vi "EV Rotator Control Editor.vi"(6 "Channel":i32=1, 8 "Calibration in":string, 9 "Hardware in":string, 10 "Setup in":string, 11 "Editor seq info":T1 {"Steps config"."Loop Info"."unit scale" items=["Log", "Lin"]; "Steps config"."Loop Info"."unit dB ref" format="%#_6p"}) -> (1 "Step name out":string="Calibration Default", 2 "Setup out":string, 3 "Sequence channels & curves out":string[](array[string]))   [LabVIEW 2012]
uses:
  custom and SC Run Seq Sub VIs.llb/editor seq info.ctl
  custom and SC Run Seq Sub VIs.llb/Steps config.ctl
panel:
  in  "Absolute mode":bool
  in  "Port name":string
  in  "Function to run":enum16{"Home", "MoveDegrees"}(ring)
  in  "Vertical angle":dbl format="%.3f"
  in  "Horizontal angle":dbl format="%.3f"
  in  "Save as":bool
  in  "save":bool
  in  "revert":bool
  in  "continue loop?":bool
  in  "cancel":bool
  in  "load":bool
  # "Reminder:  You must edit this custom step from\nwithin a sequence for it to remember your settings."
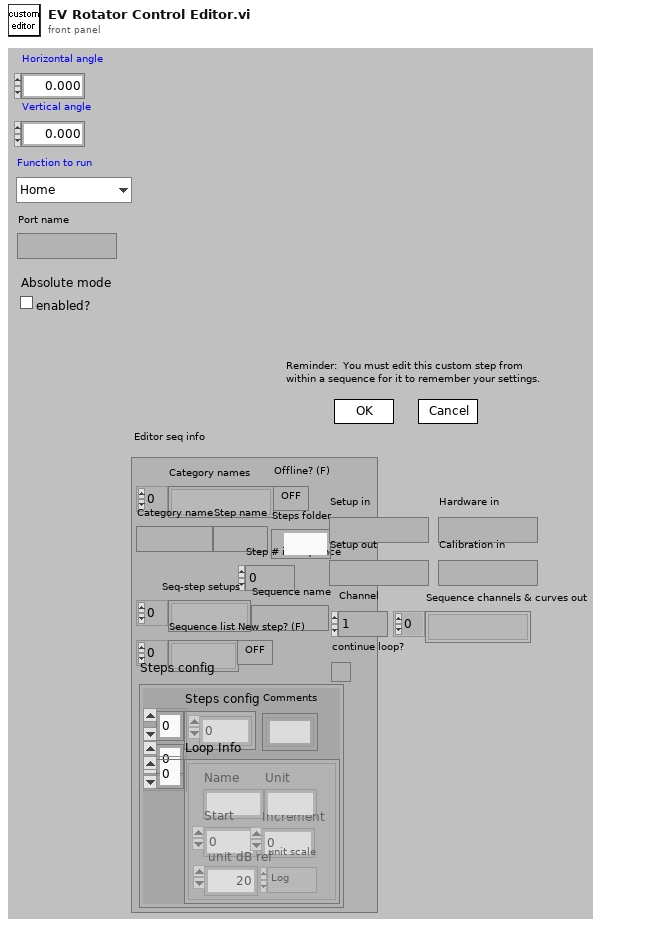
[diagram p1: front panel]
types:
  T1 = typedef "editor seq info.ctl" = cluster{"Category names":string[], "Category name":string, "Step name":string, "Step # in sequence":i32, "Seq-step setups":string[], "Sequence name":string, "Sequence list":string[], "New step? (F)":bool, "Steps config":T2, "Offline? (F)":bool, "Steps folder":path}
  T2 = typedef "Steps config.ctl" = cluster{"Steps config":i32[][], "Loop Info":cluster{"Name":string, "Start":dbl, "Increment":dbl, "Unit":string, "unit dB ref":dbl, "unit scale":u16}[], "Comments":string[]}
  T3 = cluster{"Horizontal angle":dbl, "Vertical angle":dbl, "FunctionToRun":enum16{"Home", "MoveDegrees"}, "Port name":string, "Absolute position mode":bool}
  T4 = cluster{"load":bool, "revert":bool, bool, "cancel":bool, "Save as":bool, bool, bool}
  T5 = cluster{"load":bool, "revert":bool, "save":bool, "cancel":bool, "Save as":bool, "close panel":bool, "apply":bool}
  T6 = typedef "seq step setup.ctl" = cluster{"Input Signal Channels":i32[], "Output Signal Channels":i32[], "Curves selected":string[][], "Curves generated":string[], "Step setup flat":string, "Trigger Signal Channel":i32, "Curves Generated Assumptions":cluster{"seq-setup in":string, "Relevant subset of mem list Grouping":cluster{T7[]}[]}}
  T7 = typedef "Memory List Grouping.ctl" = cluster{"item name":string, "parent":string, "Open?":bool, "Type":enum16{"item", "custom group", "auto group"}}
  T8 = typedef "data cluster.ctl" = cluster{"Name":string, "Curve":cluster{"x":dbl, "y":dbl, "z":dbl}[], "X data":T9, "Y data":T9, "Z data":T9, "X axis":u16, "Y axis":u16, "Z axis":u16, "X unit":string, "Y unit":string, "Z unit":string, "X dB ref":dbl, "Y dB ref":dbl, "Z dB ref":dbl, "single val":bool, "protected":bool, "display X":bool, "display Y":bool, "display Z":bool, "Plot Settings":cluster{"Color":u32, "Interpolation":u8, "Point Style":u8, "Line Style":u8, "Point Color":u32, "Line Width":u8, "Bar Plot Style":u8, "Fill To":i16}, "Test Info":string}
  T9 = typedef "Axis Unit Type.ctl" = u16
  T10 = typedef "waveform cluster.ctl" = cluster{"Name":string, "Waveform":cluster{"X0":dbl, "dX":dbl, "Y":sgl[]}, "X data":T9, "Y data":T9, "Y axis":T9, "X unit":string, "Y unit":string, "Y dB ref":dbl, "display Y":bool, "display X":bool, "Overload?":bool, "protected":bool, "Sqc history":string[], "Signal Channel ID":i32, "Plot Settings":cluster{"Color":u32, "Interpolation":u8, "Point Style":u8, "Line Style":u8, "Point Color":u32, "Line Width":u8, "Bar Plot Style":u8, "Fill To":i16}, "Test Info":string}
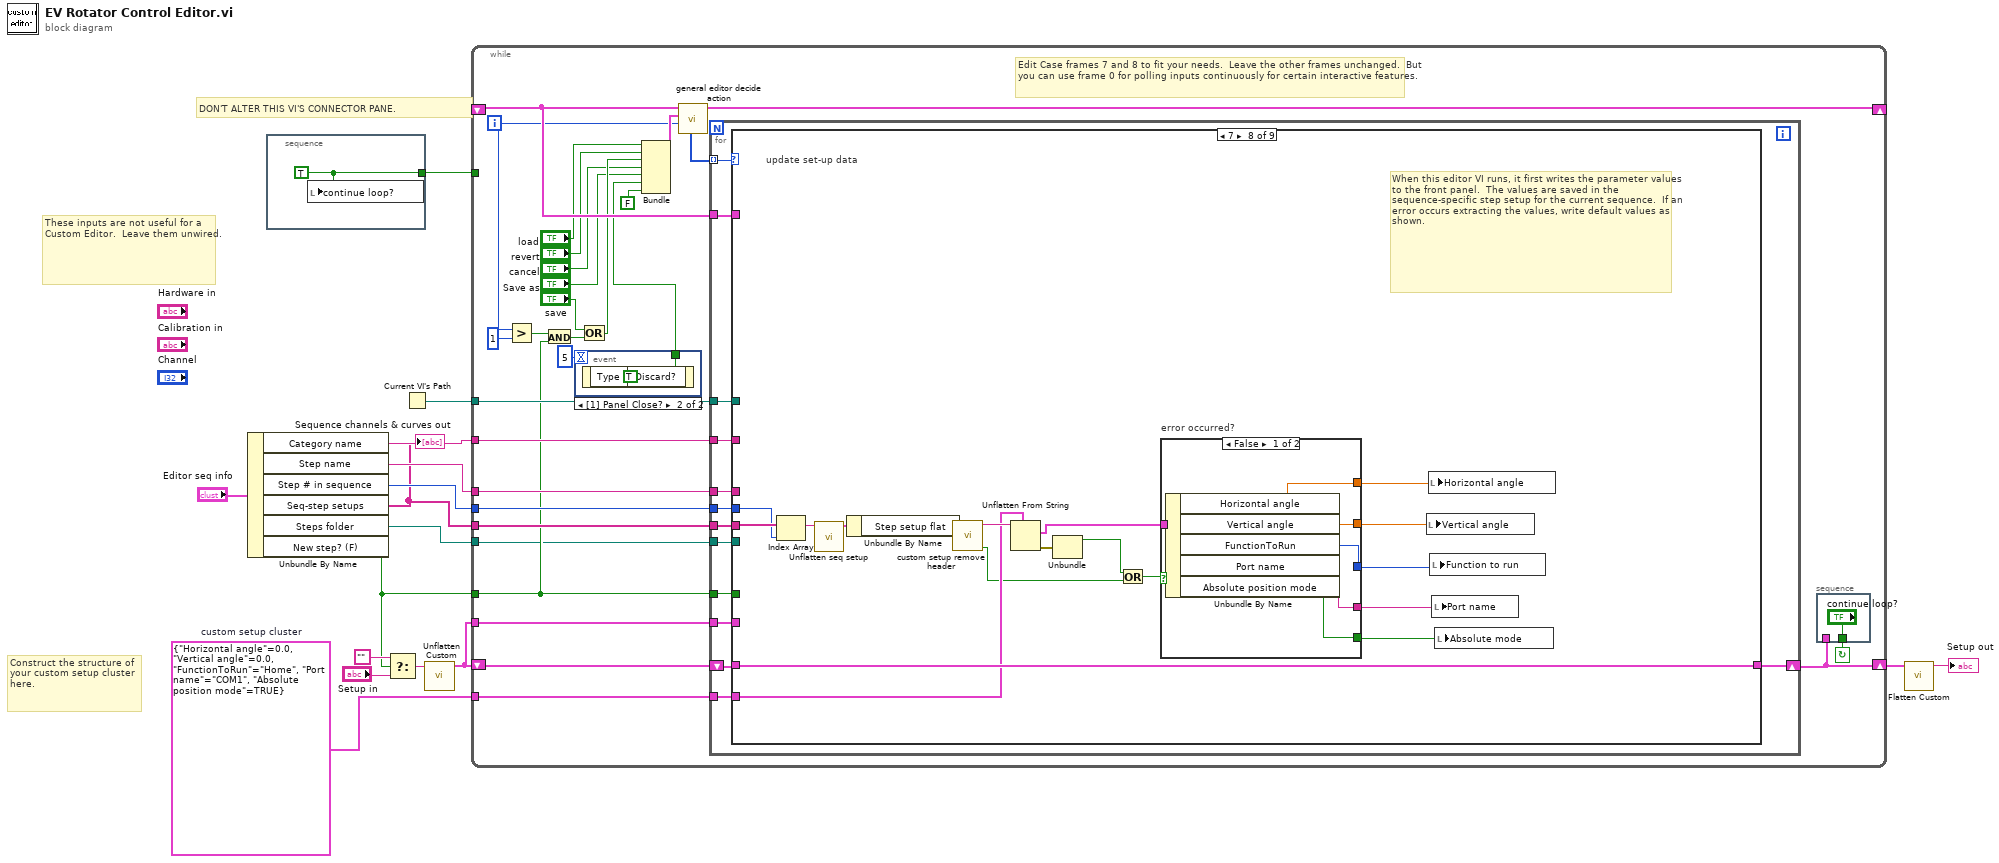
[diagram p0: block diagram]
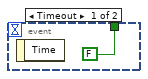
[diagram p2: hidden frame]
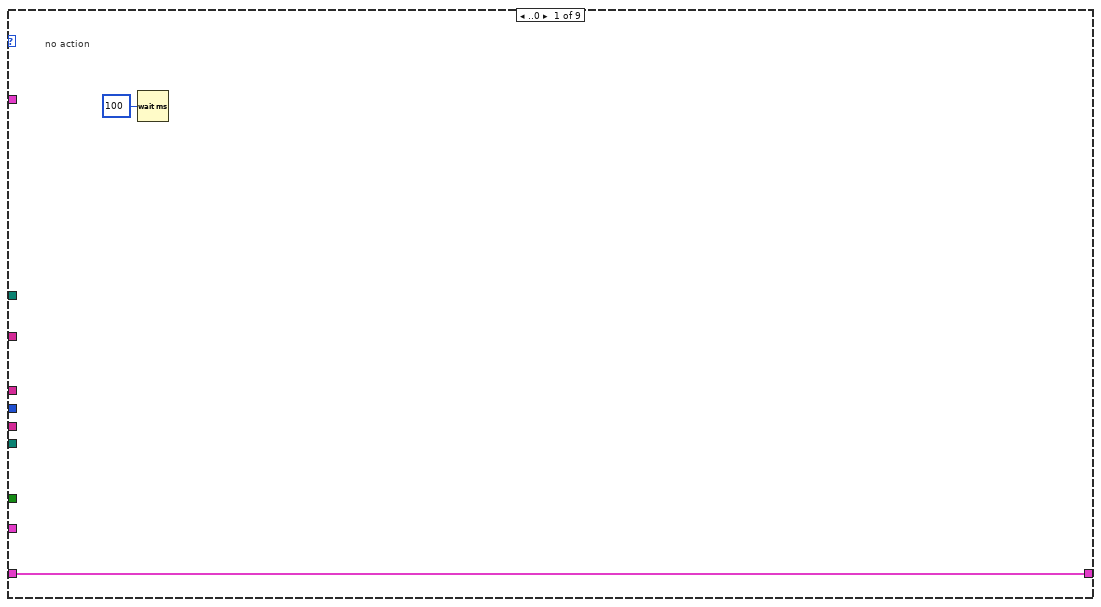
[diagram p3: hidden frame]
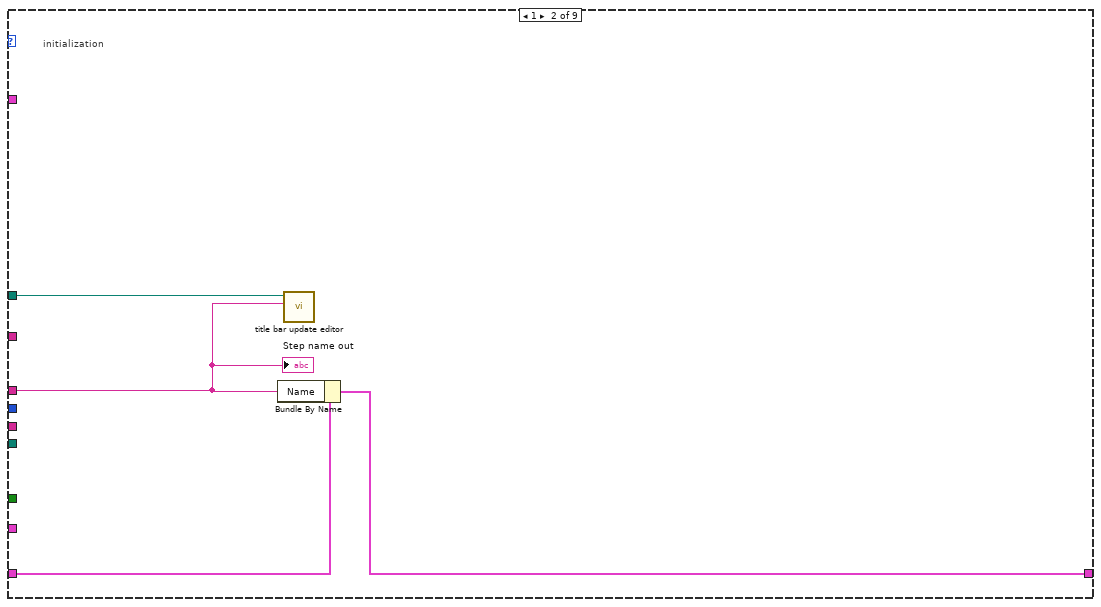
[diagram p4: hidden frame]
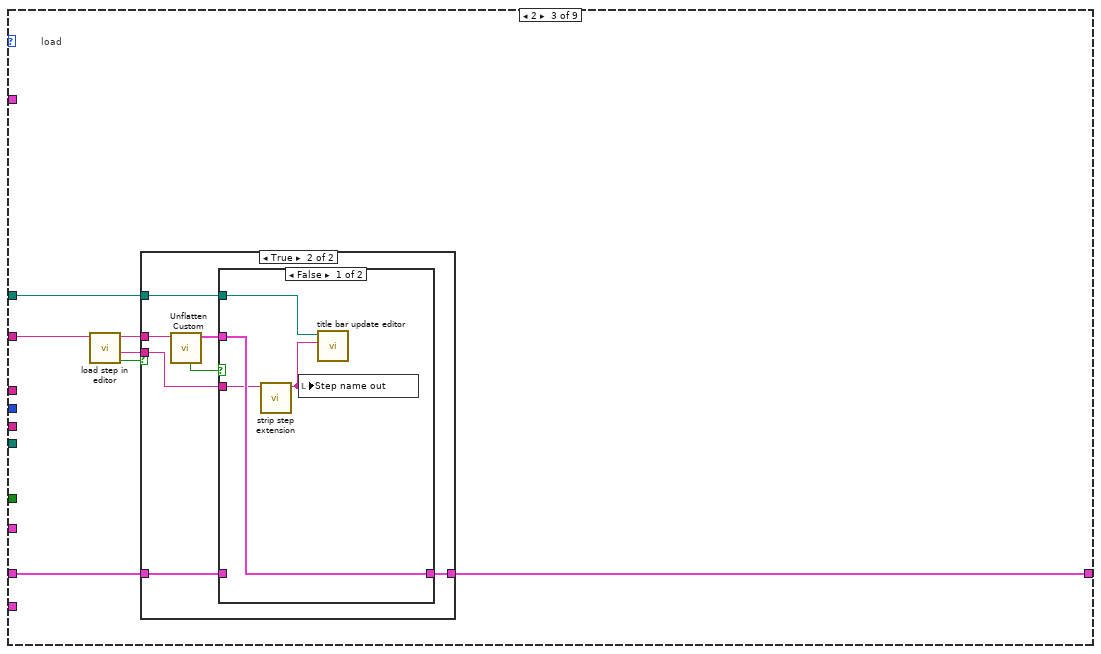
[diagram p5: hidden frame]
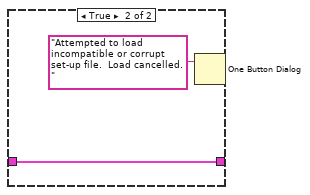
[diagram p7: hidden frame]
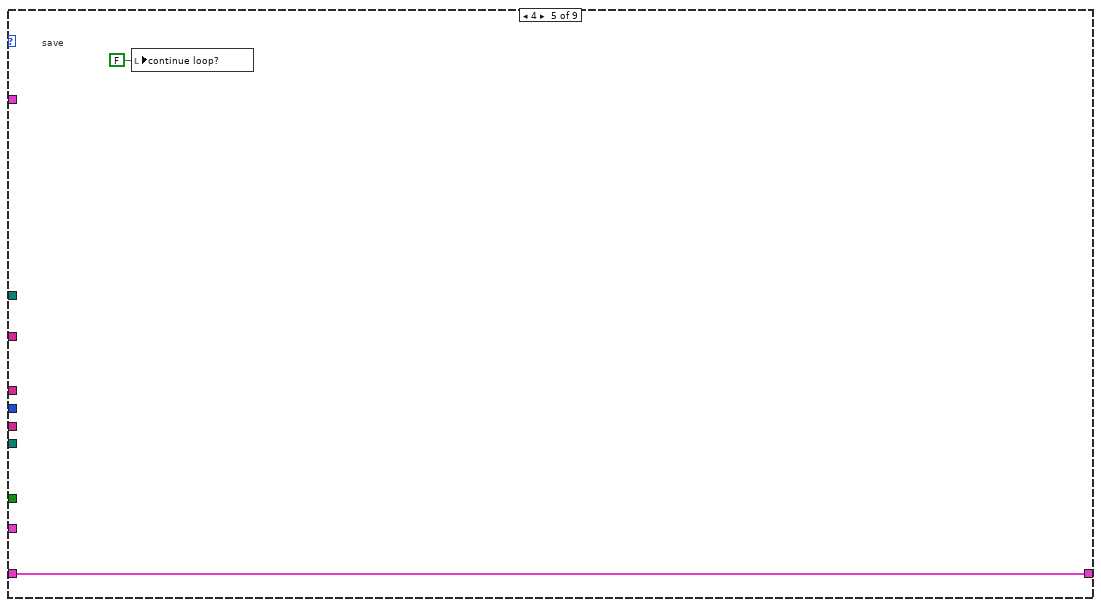
[diagram p9: hidden frame]
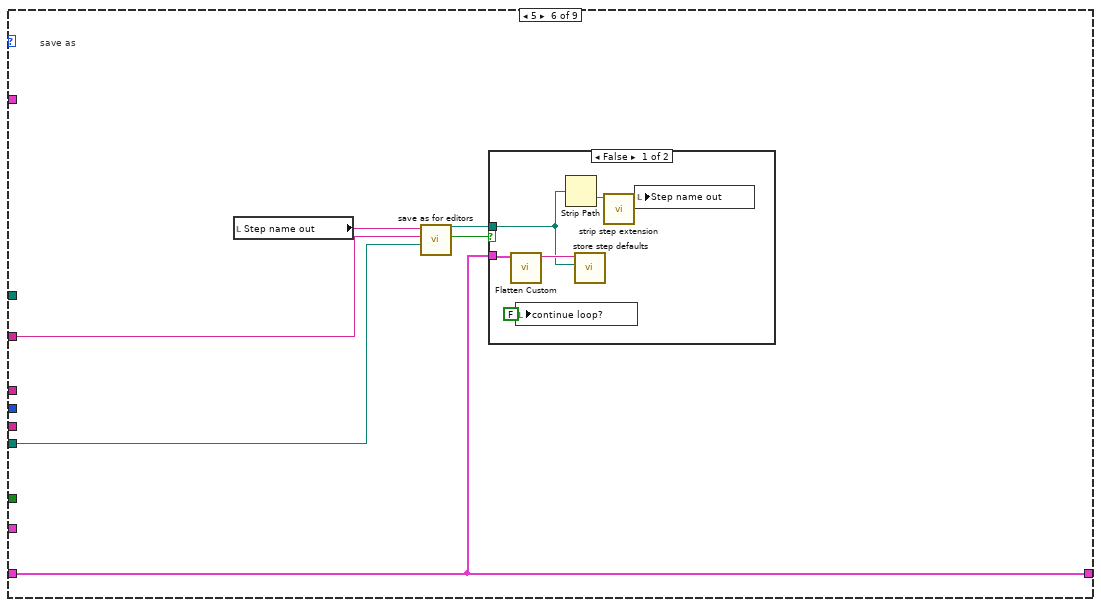
[diagram p10: hidden frame]
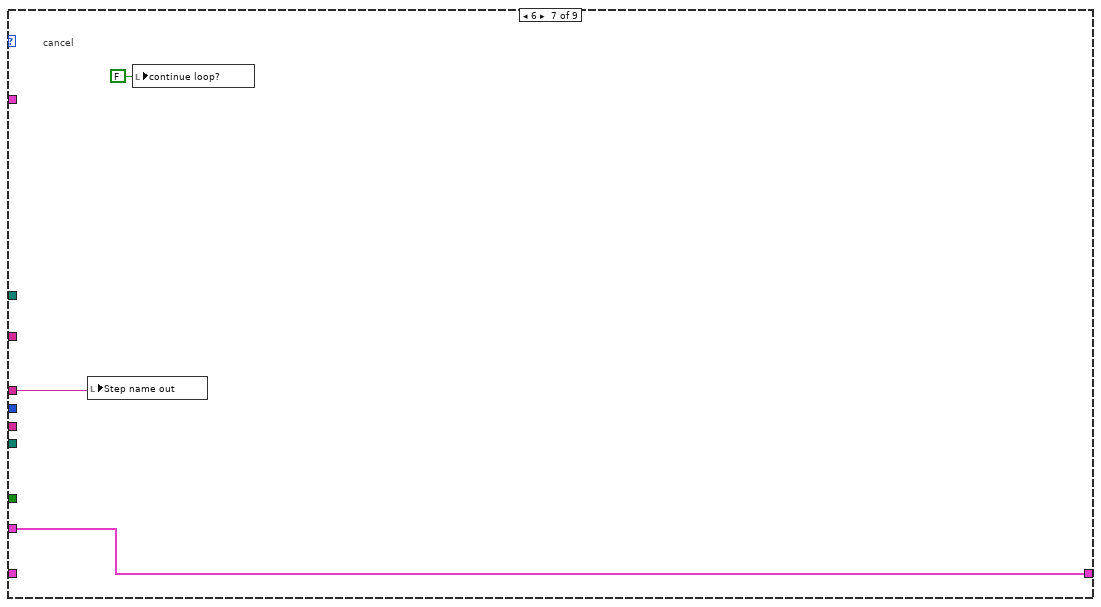
[diagram p12: hidden frame]
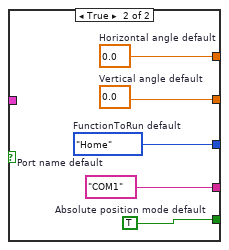
[diagram p13: hidden frame]
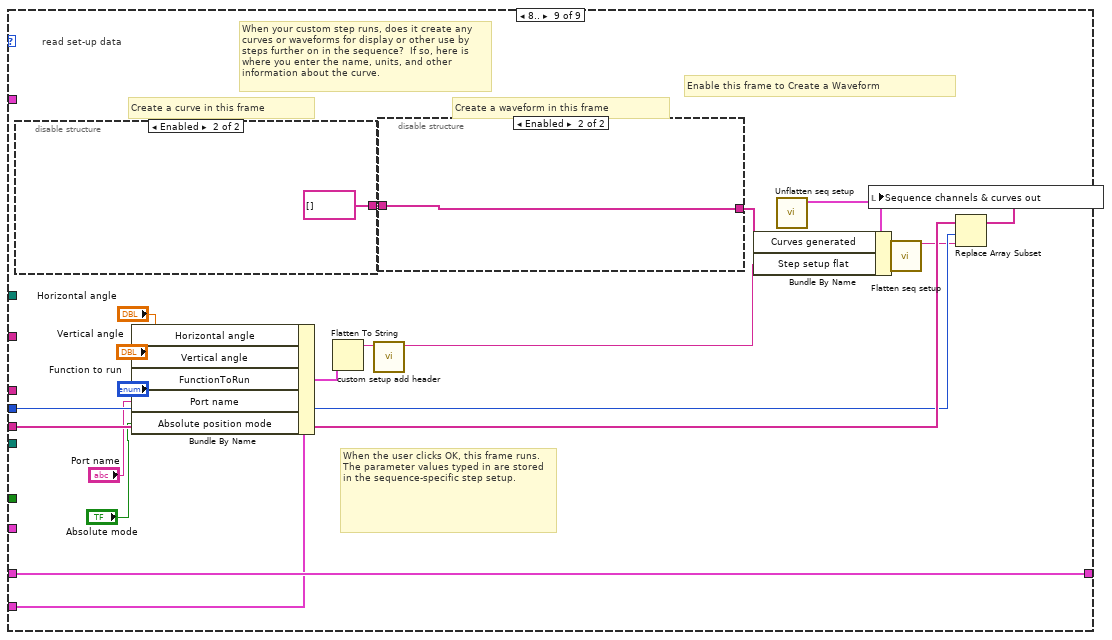
[diagram p14: hidden frame]
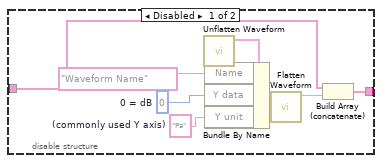
[diagram p15: hidden frame]
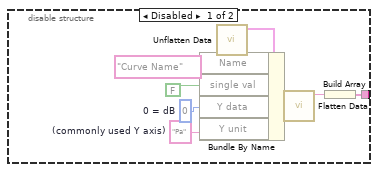
[diagram p16: hidden frame]
diagram:
  w12 = T3 {"Horizontal angle"=0.0, "Vertical angle"=0.0, "FunctionToRun"=enum."Home", "Port name"="COM1", "Absolute position mode"=TRUE}  # custom setup cluster
  # "Construct the structure of your custom setup cluster here."
  # "These inputs are not useful for a Custom Editor.  Leave them unwired."
  # "DON'T ALTER THIS VI'S CONNECTOR PANE."
  n1 = Unbundle By Name("Editor seq info") -> ("Category name"=w9:string, "Step name"=w8:string, "Step # in sequence"=w7:i32, "Seq-step setups"=w5:string[], "Steps folder"=w6:path, "New step? (F)"=w2:bool)
  "Sequence channels & curves out" <- w5
  n2 = stacked-sequence {
    tunnel: [w17] -> w10
    frame #0 {
      w17 = TRUE ("continue loop?")
      n3 = local write "continue loop?"(w17) -> ()
    }
  }
  n4 = Select(t="", s=w2, f="Setup in") -> (s? t:f=w13:string)
  n5 = Current VI's Path() -> (path=w11:path)
  n6 = call "Unflatten Custom.vi"("Unflatten Custom"=w13) -> ("Custom"=w1:cluster{"Name":string})  [unwired: 10 out]
  n7 = while {
    tunnel: w12 -> [w27]
    tunnel: w11 -> [w35]
    shift-left: w1 -> [w37]
    shift-right: [w28] -> w3
    tunnel: w1 -> [w39]
    tunnel: w2 -> [w31]
    tunnel: w5 -> [w41]
    tunnel: w7 -> [w42]
    tunnel: w8 -> [w43]
    tunnel: w9 -> [w44]
    shift-left: _ -> [w38]
    shift-right: [w46] -> _
    tunnel: w6 -> [w24]
    tunnel: w10 -> [_]
    i -> [w34]
    stop <- w40 continue-if-true
    # "Edit Case frames 7 and 8 to fit your needs.  Leave the other frames unchanged.  But you can use frame 0 for polling inputs continuously for certain interactive features."
    n8 = Greater?(x=w34, y=1) -> (0:w32:bool)
    n9 = And(x=w32, y=w31) -> (x .and. y?=w30:bool)
    n10 = event shown="[1] Panel Close?" {
      selector: _ -> [_ _]
      dyn-events: _ -> [_ _]
      timeout: 5 -> [_ _]
      tunnel: [FALSE w48] -> w26
      event Timeout {
        n11 = event-data() -> ()  [unwired: 2 out]
      }
      event Panel Close? {
        w48 = TRUE
        n12 = event-data() -> ()  [unwired: 2 out]
        n13 = event-data("Discard?"=w48) -> ()  [unwired: 1 in, 1 out]
      }
    }
    n14 = Or(x="save", y=w30) -> (x .or. y?=w29:bool)
    n15 = Bundle("load"="load", "revert"="revert", w29, "cancel"="cancel", "Save as"="Save as", w26, FALSE) -> (w36:T4)  [unwired: 1 out]
    n16 = call "general editor decide action.vi"("Iteration"=w34, "Polled cluster"=w36, "Old cluster"=w38) -> ("actions array"=w45:i32[], "New cluster"=w46:T5)  [unwired: 1 in, 6 out]
    n17 = for {
      tunnel: w38 -> [w62]
      tunnel: w39 -> [w61]
      tunnel: w31 -> [w60]
      tunnel: w41 -> [w59]
      tunnel: w42 -> [w58]
      tunnel: w43 -> [w57]
      tunnel: w44 -> [w56]
      tunnel: w45 -> [w55] mode=indexing
      shift-right: [w53] -> w28
      shift-left: w37 -> [w54]
      tunnel: w35 -> [w52]
      tunnel: w27 -> [w51]
      tunnel: w24 -> [w50]
      n18 = case shown="7" w55 {
        tunnel: w56 -> [_ _ w71 _ _ w95 _ _ _]
        tunnel: w57 -> [_ w65 _ _ _ _ w105 _ _]
        tunnel: w58 -> [_ _ _ _ _ _ _ w122 w151]
        tunnel: w59 -> [_ _ _ _ _ _ _ w123 w152]
        tunnel: w60 -> [_ _ _ _ _ _ _ _ _]
        tunnel: w61 -> [_ _ _ w90 _ _ w106 _ _]
        tunnel: [w63 w68 w75 w90 w91 w98 w106 w125 w148] -> w53
        tunnel: w54 -> [w63 w67 w74 _ w91 w98 _ w125 w148]
        tunnel: w62 -> [_ _ _ _ _ _ _ _ _]
        tunnel: w52 -> [_ w66 w69 _ _ _ _ _ _]
        tunnel: w51 -> [_ _ _ _ _ _ _ w118 w145]
        tunnel: w50 -> [_ _ _ _ _ w93 _ _ _]
        frame ..0 {
          # "no action"
          n19 = Wait (ms)(milliseconds to wait=u32 100) -> ()  [unwired: 1 out]
        }
        frame 1 {
          # "initialization"
          n20 = Bundle By Name(cluster=w67, "Name"=w65) -> (w68:cluster{"Name":string})
          n21 = call "title bar update editor.vi"("Step name"=w65, "Editor VI path"=w66) -> ()  [unwired: 10 out]
          "Step name out" <- w65
        }
        frame 2 {
          # "load"
          n22 = call "load step in editor.vi"("Category name"=w71) -> ("Not canceled?"=w72:bool, "New step name (with ext.)"=w70:string, "Flat step set-up"=w73:string)  [unwired: 1 in, 7 out]
          n23 = case shown="True" w72 {
            tunnel: w73 -> [_ w83]
            tunnel: [w76 w81] -> w75
            tunnel: w74 -> [w76 w80]
            tunnel: w70 -> [_ w78]
            tunnel: w69 -> [_ w77]
            frame False {
            }
            frame True {
              n24 = call "Unflatten Custom.vi"("Unflatten Custom"=w83) -> ("Custom"=w79:cluster{"Name":string}, "Error?"=w82:bool)  [unwired: 9 out]
              n25 = case shown="False" w82 {
                tunnel: [w87 w89] -> w81
                tunnel: w80 -> [_ w89]
                tunnel: w79 -> [w87 _]
                tunnel: w78 -> [w86 _]
                tunnel: w77 -> [w85 _]
                frame False {
                  n26 = call "strip step extension.vi"("Step name w/ extension"=w86) -> ("Step name (base)"=w84:string)  [unwired: 1 in, 9 out]
                  n27 = local write "Step name out"(w84) -> ()
                  n28 = call "title bar update editor.vi"("Step name"=w84, "Editor VI path"=w85) -> ()  [unwired: 10 out]
                }
                frame True {
                  n29 = One Button Dialog(message="Attempted to load incompatible or corrupt set-up file.  Load cancelled.") -> ()  [unwired: 2 out]
                }
              }
            }
          }
        }
        frame 3 {
          # "revert"
        }
        frame 4 {
          # "save"
          n30 = local write "continue loop?"(FALSE ("continue loop?")) -> ()
        }
        frame 5 {
          # "save as"
          n31 = local read "Step name out"() -> (w94:string)
          n32 = call "save as for editors.vi"("Steps Folder (gbl if empty)"=w93, "Category name"=w95, "Step name"=w94) -> ("Canceled"=w96:bool, "File path chosen"=w97:path)  [unwired: 3 in, 4 out]
          n33 = case shown="False" w96 {
            tunnel: w97 -> [w100 _]
            tunnel: w98 -> [w103 _]
            frame False {
              n34 = call "Flatten Custom.vi"("Custom"=w103) -> ("Custom flattened"=w104:string)  [unwired: 10 out]
              n35 = local write "continue loop?"(FALSE ("continue loop?")) -> ()
              n36 = Strip Path(path=w100) -> (name=w101:string)  [unwired: 1 out]
              n37 = call "store step defaults.vi"("Set-up file"=w100, "Flat step set-up"=w104) -> ()  [unwired: 4 in, 6 out]
              n38 = call "strip step extension.vi"("Step name w/ extension"=w101) -> ("Step name (base)"=w99:string)  [unwired: 1 in, 9 out]
              n39 = local write "Step name out"(w99) -> ()
            }
            frame True {
            }
          }
        }
        frame 6 {
          # "cancel"
          n40 = local write "Step name out"(w105) -> ()
          n41 = local write "continue loop?"(FALSE ("continue loop?")) -> ()
        }
        frame 7 {
          # "When this editor VI runs, it first writes the parameter values to the front panel.  The values are saved in the sequence-specific step setup for the current sequence.  If an error occurs extracting the values, write default values as shown."
          # "update set-up data"
          n42 = Index Array(array=w123, index=w122) -> (element=w124:string)
          n43 = call "Unflatten seq setup.vi"("Unflatten seq setup"=w124) -> ("Sequence-specific step set-up"=w121:T6)  [unwired: 3 in, 7 out]
          n44 = Unbundle By Name(w121) -> ("Step setup flat"=w120:string)
          n45 = call "custom setup remove header.vi"("Output from 'Step setup flat' of seq-setup structure"=w120) -> ("Error?"=w117:bool, "Flattened custom step setup cluster"=w119:string)  [unwired: 9 out]
          n46 = Unflatten From String(type=w118, binary string=w119) -> (value=w114:T3, error out=w111:errorcluster)  [unwired: 1 in, 3 out]
          n47 = Unbundle(w111) -> ("status"=w116:bool)  [unwired: 2 out]
          n48 = Or(x=w116, y=w117) -> (x .or. y?=w115:bool)
          n49 = case "error occurred?" shown="False" w115 {
            tunnel: w114 -> [w131 _]
            tunnel: [w130 w135] -> w113
            tunnel: [w129 w136] -> w112
            tunnel: [w127 w134] -> w110
            tunnel: [w128 w133] -> w109
            tunnel: [w126 w132] -> w108
            frame False {
              n50 = Unbundle By Name(w131) -> ("Horizontal angle"=w129:dbl, "Vertical angle"=w130:dbl, "FunctionToRun"=w127:enum16{"Home", "MoveDegrees"}, "Port name"=w128:string, "Absolute position mode"=w126:bool)
            }
            frame True {
              w132 = TRUE  # Absolute position mode default
              w133 = "COM1"  # Port name default
              w134 = enum16{"Home", "MoveDegrees"}."Home"  # FunctionToRun default
              w135 = 0.0  # Vertical angle default
              w136 = 0.0  # Horizontal angle default
            }
          }
          n51 = local write "Vertical angle"(w113) -> ()
          n52 = local write "Horizontal angle"(w112) -> ()
          n53 = local write "Function to run"(w110) -> ()
          n54 = local write "Port name"(w109) -> ()
          n55 = local write "Absolute mode"(w108) -> ()
        }
        frame 8.. {
          # "Enable this frame to Create a Waveform"
          # "Create a waveform in this frame"
          # "Create a curve in this frame"
          # "When your custom step runs, does it create any curves or waveforms for display or other use by steps further on in the sequence?  If so, here is where you enter the name, units, and other information about the curve."
          # "When the user clicks OK, this frame runs.  The parameter values typed in are stored in the sequence-specific step setup."
          # "read set-up data"
          n56 = disable-structure shown="Enabled" {
            disable-tunnel: [w164 string[] []] -> w143
            frame Disabled {
              w165 = "Pa"  # (commonly used Y axis)
              w169 = u16 0  # 0 = dB
              n57 = call "Unflatten Data.vi"() -> ("Datum"=w168:T8)  [unwired: 1 in, 10 out]
              n58 = Bundle By Name(cluster=w168, "Name"="Curve Name", "single val"=FALSE, "Y data"=w169, "Y unit"=w165) -> (w166:T8)
              n59 = call "Flatten Data.vi"("Datum"=w166) -> ("Data flattened"=w171:string)  [unwired: 10 out]
              n60 = Build Array(w171) -> (w164:string[])
            }
            frame Enabled {
            }
          }
          n61 = Bundle By Name(cluster=w145, "Horizontal angle"="Horizontal angle", "Vertical angle"="Vertical angle", "FunctionToRun"="Function to run", "Port name"="Port name", "Absolute position mode"="Absolute mode") -> (w144:T3)
          n62 = Flatten To String(anything=w144) -> (data string=w146:string)  [unwired: 1 in, 4 out]
          n63 = call "custom setup add header.vi"("Flattened custom step setup cluster"=w146) -> ("Input to 'Step setup flat' of seq-setup structure"=w147:string)  [unwired: 1 in, 9 out]
          n64 = disable-structure shown="Enabled" {
            disable-tunnel: [w157 w163] -> w142
            disable-tunnel: w143 -> [w155 w163]
            frame Disabled {
              w158 = "Pa"  # (commonly used Y axis)
              w161 = u16 0  # 0 = dB
              n65 = call "Unflatten Waveform.vi"() -> ("Unflattened Waveform"=w160:T10)  [unwired: 9 in, 2 out]
              n66 = Bundle By Name(cluster=w160, "Name"="Waveform Name", "Y data"=w161, "Y unit"=w158) -> (w156:T10)
              n67 = call "Flatten Waveform.vi"("Waveform"=w156) -> ("Waveform flattened"=w162:string)  [unwired: 10 in]
              n68 = Build Array (concatenate)(w155, w162) -> (w157:string[])
            }
            frame Enabled {
            }
          }
          n69 = call "Unflatten seq setup.vi"() -> ("Sequence-specific step set-up"=w154:T6)  [unwired: 4 in, 7 out]
          n70 = Bundle By Name(cluster=w154, "Curves generated"=w142, "Step setup flat"=w147) -> (w153:T6)
          n71 = call "Flatten seq setup.vi"("Sequence-specific step set-up"=w153) -> ("Seq setup flattened"=w150:string)  [unwired: 10 out]
          n72 = Replace Array Subset(array=w152, new element=w150, index=w151) -> (w149:string[])
          n73 = local write "Sequence channels & curves out"(w149) -> ()
        }
      }
    }
    n74 = stacked-sequence {
      tunnel: ["continue loop?"] -> w40
      tunnel: w28 -> [_]
      frame #0 {
      }
    }
  }
  n75 = call "Flatten Custom.vi"("Custom"=w3) -> ("Custom flattened"=→"Setup out":string)  [unwired: 10 out]
